vi "FileoutTest.vi"() -> ()   [LabVIEW 2018]
uses:
  <vilib>/Platform/TimedLoop/XDataNode/timing_clust.ctl
  <vilib>/Platform/TimedLoop/XDataNode/nitl_modes.ctl
  <vilib>/Platform/TimedLoop/XDataNode/wakeup.ctl
  <vilib>/express/express signal manip/GetorSetDDTAttributes/Shared VIs/XDimension.ctl
  21fbdac2-0775-4e8d-9e09-8832f3958a18.vi
  <vilib>/express/express signal manip/GetorSetDDTAttributes/Shared VIs/XDimension Enum to String.vi
  <vilib>/express/express shared/transition.llb/Dynamic To Waveform Array.vi
  <vilib>/express/express signal manip/GetorSetDDTAttributes/Set DDT Attributes/SetT0.vi
  <vilib>/express/express signal manip/GetorSetDDTAttributes/Set DDT Attributes/sub Set StartTimeStamp.vi
  <vilib>/express/express shared/transition.llb/Waveform Array To Dynamic.vi
  <vilib>/platform/TimedLoop/XDataNode/XDataNode.xnode
  <vilib>/express/express signal manip/GetorSetDDTAttributes/Set DDT Attributes/Set DDT Properties.xnode
  <vilib>/Platform/TimedLoop/XDataNode/XDNodeRunTimeDep.lvlib
  <vilib>/express/express signal manip/GetorSetDDTAttributes/Shared VIs/GetSetShared.lvlib
  <vilib>/express/express signal manip/GetorSetDDTAttributes/Set DDT Attributes/Set DDT Attributes.lvlib
panel:
  out "# elements in queue":i32
  out "RecState Out":T1(ring)
  in  "Filepath":path=path "C:/LPLDocs/log.lvm"
  in  "Record":bool
  in  "RecState":T1(ring)
  out "Cycle Count":i32
  # "Fileout Unit Test Procedures:\n\nReturn to the default position after each test\n\nSetup:\nNone\n\n1) Run and activate Record\n        Verify that the log file at the specified Filepath contains correct X column data for the duration of the recording\n        Verify that the log file contains the correct span of Cycle Counts in the TestSignal column\n2) Run and activate record.\n        Verify that RecState out reads Normal if # elements of queue is positive and Ready for New File when it is zero\n        Set RecState to Ready for New File\n        Verify that RecState out reads Normal if # elements of queue is positive and Ready for New File when it is zero\n        Wait 1 minute, then set RecState to New File, record the value of CycleCount at this point\n        Verify that RecState out reads Normal if # elements of queue is positive and Ready for New File when it is zero\n        Stop recording\n        Verify that two logs have been created, and the second log begins at the CycleCount above"
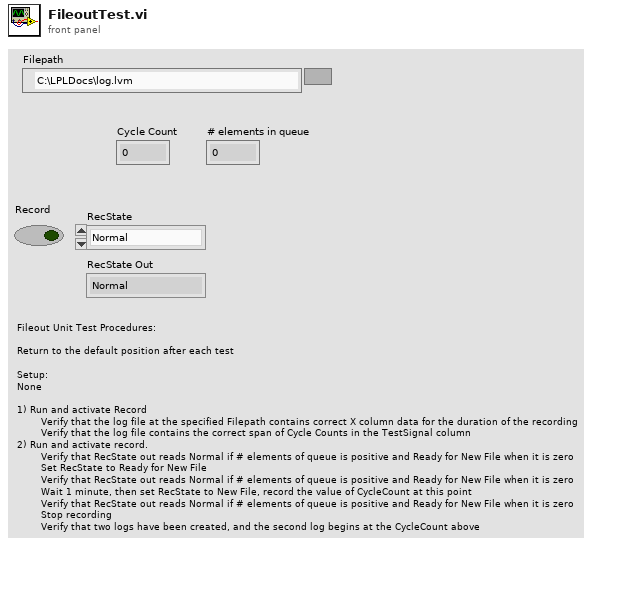
[diagram p1: front panel]
types:
  T1 = enum16{"Normal", "Overdrive", "Ready for Overdrive End", "Ready for new file", "New file"}
  T2 = typedef "XDNodeRunTimeDep.lvlib/timing_clust.ctl" = cluster{"Expected End [f-1]":u64, "Actual End [f-1]":u64, "Finished Late? [f-1]":bool, "Expected End [i-1]":u64, "Actual End [i-1]":u64, "Finished Late? [i-1]":bool, "Expected Start [i]":u64, "Actual Start [i]":u64, "Expected Start [f]":u64, "Actual Start [f]":u64, "Source Name":string, "Structure Name":string, "Period":i64, "Deadline":i64, "Offset":i64, "Start":i64, "Priority":i32, "Timeout":i32, "Mode":T3, "Wakeup Reason":T4, "Error":errorcluster, "Source Type":string, "Secondary Source Type":string, "Global End Time":u64, "Global Start Time":u64, "Frame Duration":u64, "Iteration Duration":u64, "Assigned CPU":i32, "I/O Scan Engine Mode":u32}
  T3 = typedef "XDNodeRunTimeDep.lvlib/nitl_modes.ctl" = enum32{"No Change", "Process missed periods, maintain original phase", "Discard missed periods, maintain original phase", "Process missed periods, ignore original phase", "Discard missed periods, ignore original phase"}
  T4 = typedef "XDNodeRunTimeDep.lvlib/wakeup.ctl" = enum32{"Normal", "Aborted", "Asynchronous wakeup", "Timing source error", "Timed loop error", "Timeout"}
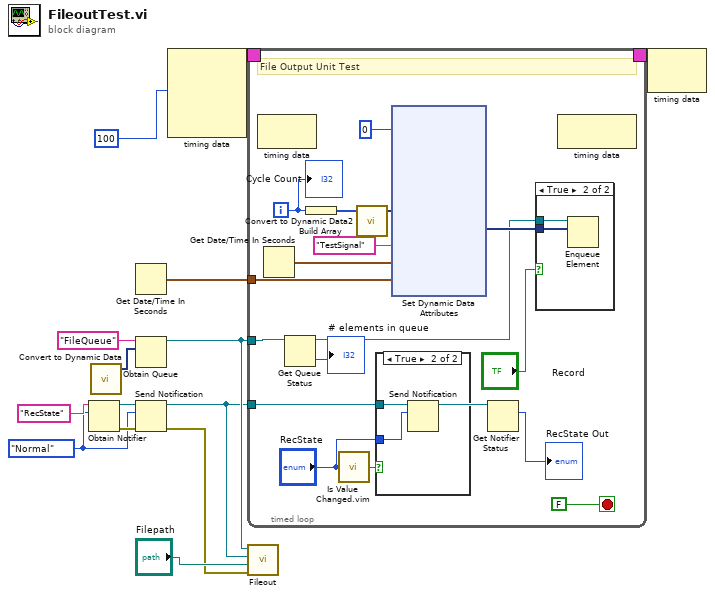
[diagram p0: block diagram]
diagram:
  w9 = T1."Normal" ("RecState")
  n1 = Obtain Notifier(name (unnamed)="RecState", notification data type=w9) -> (notifier out=w10:refnum<notifier>, error out=w11:errorcluster)  [unwired: 2 in, 1 out]
  n2 = call "Convert to Dynamic Data"() -> ("Dynamic Data Type"=w13:dynamicdata)  [unwired: 4 in]
  n3 = Get Date/Time In Seconds() -> (seconds since 1Jan1904=w8:timestamp)
  n4 = Obtain Queue(name (unnamed)="FileQueue", element data type=w13) -> (queue out=w4:refnum<queue>)  [unwired: 3 in, 2 out]
  n5 = Send Notification(notification=w9, notifier=w10, error in (no error)=w11) -> (notifier out=w3:refnum<notifier>, error out=w1:errorcluster)
  n6 = node-c288(i64 100 ("Period")) -> (w7:T2)  [unwired: 3 in]
  n7 = timed-loop {
    tunnel: w8 -> [w30]
    tunnel: w4 -> [w22]
    tunnel: w3 -> [w19]
    timing: w7 -> [_]
    timing-out: [_] -> w6
    i -> [w28]
    stop <- FALSE stop-if-true
    # "File Output Unit Test"
    n8 = node-c288() -> ()  [unwired: 1 in, 1 out]
    n9 = Get Date/Time In Seconds() -> (seconds since 1Jan1904=w29:timestamp)
    n10 = Get Queue Status(queue=w22) -> (queue out=w17:refnum<queue>, # elements in queue=→"# elements in queue":i32)  [unwired: 2 in, 6 out]
    n11 = Build Array(w28) -> (w27:i32[])
    n12 = call "Is Value Changed.vim"("value"="RecState") -> ("changed or first call?"=w25:bool)
    n13 = call "Convert to Dynamic Data2"("Array"=w27) -> ("Dynamic Data Type"=w26:dynamicdata)  [unwired: 3 in]
    n14 = case shown="True" w25 {
      tunnel: "RecState" -> [_ w36]
      tunnel: w19 -> [_ w37]
      frame False {
      }
      frame True {
        n15 = Send Notification(notification=w36, notifier=w37) -> ()  [unwired: 1 in, 2 out]
      }
    }
    n16 = xnode "Set Dynamic Data Attributes"("Signals In"=w26, "Signal Name"="TestSignal", "Timestamp"=w29, "Start Timestamp"=w30, "Signal Index"=0) -> ("Signals Out"=w23:dynamicdata)  [unwired: 2 in, 1 out]
    n17 = Get Notifier Status(notifier=w19) -> (current notification=→"RecState Out":T1)  [unwired: 1 in, 4 out]
    n18 = case shown="True" "Record" {
      tunnel: w23 -> [_ w33]
      tunnel: w17 -> [_ w32]
      frame False {
      }
      frame True {
        n19 = Enqueue Element(queue=w32, element=w33) -> ()  [unwired: 2 in, 3 out]
      }
    }
    n20 = node-c288() -> ()  [unwired: 1 in, 1 out]
    "Cycle Count" <- w28
  }
  n21 = call "Fileout.vi"("error in (no error)"=w1, "Filepath"="Filepath", "RecState"=w3, "Logging Queue"=w4) -> ()  [unwired: 7 in, 1 out]
  n22 = node-c288(w6) -> ()  [unwired: 1 out]
